vi "Read Section.vi"(8 "Error In":errorcluster, 10 "Section":string, 11 "Path":path) -> (0 "Error Out":errorcluster, 2 "Data":string)   [LabVIEW 2020, in "Configit.lvlib"]
uses:
  Configit.lvlib
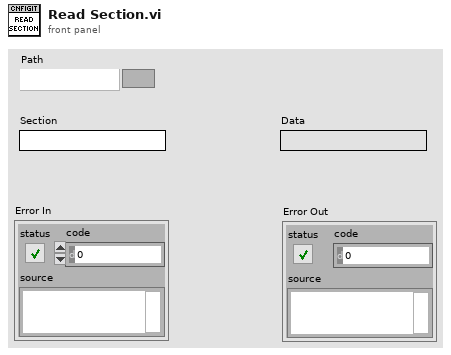
[diagram p1: front panel]
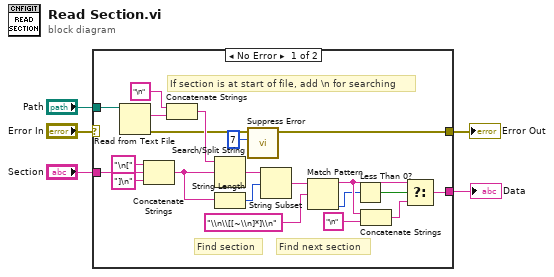
[diagram p0: block diagram]
diagram:
  n1 = case shown="No Error" "Error In" {
    selector: "Error In" -> [_ w27]
    tunnel: "Path" -> [w9 _]
    tunnel: [w8 w27] -> w4
    tunnel: "Section" -> [w7 _]
    tunnel: [w6 _] -> w2
    frame No Error {
      # "Find next section"
      # "Find section"
      # "If section is at start of file, add \\n for searching"
      n2 = Read from Text File(file (use dialog)=w9) -> (text=w23:string, error out=w11:errorcluster)  [unwired: 1 in, 4 out]
      n3 = Concatenate Strings("\n[" ("string"), w7, "]\n" ("string")) -> (w18:string)
      n4 = Concatenate Strings("\n" ("string"), w23) -> (w22:string)
      n5 = Search/Split String(string=w22, search string/char (-)=w18) -> (match + rest of string=w20:string)  [unwired: 1 in, 2 out]
      n6 = String Length(string=w18) -> (length=w17:i32)
      n7 = call "Suppress Error.vi"("Error Code"=7, "Error In"=w11) -> ("Error Out"=w8:errorcluster)  [unwired: 4 in, 1 out]
      n8 = String Subset(string=w20, offset (0)=w17) -> (substring=w19:string)  [unwired: 1 in]
      n9 = Match Pattern(string=w19, regular expression="\\n\\[[~\\n]*]\\n") -> (before substring=w15:string, offset past match=w13:i32)  [unwired: 3 out]
      n10 = Less Than 0?(x=w13) -> (x < 0?=w12:bool)
      n11 = Concatenate Strings(w15, "\n" ("string")) -> (w16:string)
      n12 = Select(t=w15, s=w12, f=w16) -> (s? t:f=w6:string)
    }
    frame Error {
    }
  }
  "Error Out" <- w4
  "Data" <- w2
